vi "Helper Loop.vi"(8 "error in (no error)":errorcluster, 11 "Helper Loop in":refnum<class "Helper Loop.lvclass">) -> (0 "error out":errorcluster, 3 "Helper Loop out":refnum<class "Helper Loop.lvclass">)   [LabVIEW 2024, in "Helper Loop.lvlib" / "Helper Loop.lvclass"]
uses:
  Helper Loop.lvclass
  Helper Loop.lvclass/Helper Loop.ctl
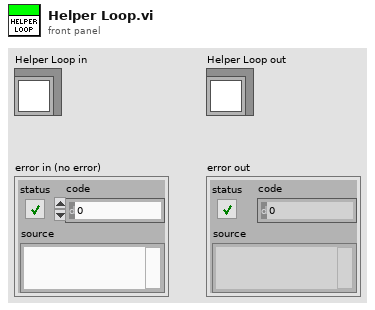
[diagram p1: front panel]
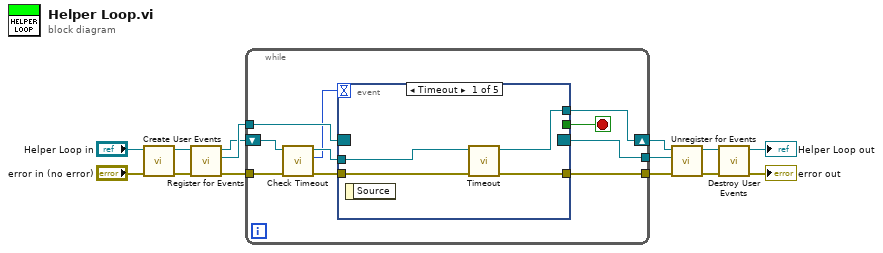
[diagram p0: block diagram]
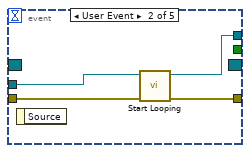
[diagram p2: hidden frame]
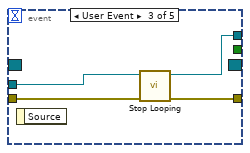
[diagram p3: hidden frame]
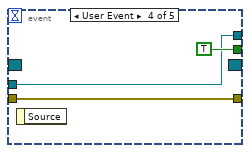
[diagram p4: hidden frame]
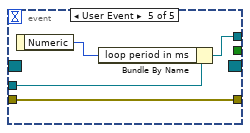
[diagram p5: hidden frame]
diagram:
  n1 = call-dynamic "Create User Events.vi"("error in (no error)"="error in (no error)", "Helper Loop in"="Helper Loop in") -> ("error out"=w11:errorcluster, "Helper Loop out"=w12:refnum<class "Helper Loop.lvclass">)  [unwired: 8 in]
  n2 = call-dynamic "Register for Events.vi"("error in (no error)"=w11, "Helper Loop in"=w12) -> ("error out"=w8:errorcluster, "event registration refnum"=w10:refnum<event-registration>, "Helper Loop out"=w9:refnum<class "Helper Loop.lvclass">)  [unwired: 7 in]
  n3 = while {
    shift-right: [w24] -> w5
    shift-left: w9 -> [w19]
    tunnel: w10 -> [w20]
    tunnel: [w22] -> w2
    tunnel: w8 -> [w18]
    tunnel: [w21] -> w1
    stop <- w23 stop-if-true
    n4 = call-dynamic "Check Timeout.vi"("error in (no error)"=w18, "Helper Loop in"=w19) -> ("error out"=w15:errorcluster, "timeout"=w16:i32, "Helper Loop out"=w17:refnum<class "Helper Loop.lvclass">)  [unwired: 7 in]
    n5 = event shown="[0] Timeout" {
      selector: w20 -> [_ _ _ _ _]
      dyn-events: [_ _ _ _ _] -> w21
      timeout: w16 -> [_ _ _ _ _]
      tunnel: [w27 w29 w33 w38 w41] -> w24
      tunnel: w17 -> [w28 w32 w36 w38 w43]
      tunnel: [_ _ _ TRUE _] -> w23
      tunnel: [w26 w30 w34 w37 w40] -> w22
      tunnel: w15 -> [w25 w31 w35 w37 w40]
      event Timeout {
        n6 = event-data() -> ()  [unwired: 1 in, 1 out]
        n7 = call-dynamic "Timeout.vi"("error in (no error)"=w25, "Helper Loop in"=w28) -> ("error out"=w26:errorcluster, "Helper Loop out"=w27:refnum<class "Helper Loop.lvclass">)  [unwired: 8 in]
      }
      event User Event {
        n8 = event-data() -> ()  [unwired: 1 in, 1 out]
        n9 = call-dynamic "Start Looping.vi"("error in (no error)"=w31, "Helper Loop in"=w32) -> ("error out"=w30:errorcluster, "Helper Loop out"=w29:refnum<class "Helper Loop.lvclass">)  [unwired: 8 in]
      }
      event User Event {
        n10 = event-data() -> ()  [unwired: 1 in, 1 out]
        n11 = call-dynamic "Stop Looping.vi"("error in (no error)"=w35, "Helper Loop in"=w36) -> ("error out"=w34:errorcluster, "Helper Loop out"=w33:refnum<class "Helper Loop.lvclass">)  [unwired: 8 in]
      }
      event User Event {
        n12 = event-data() -> ()  [unwired: 1 in, 1 out]
      }
      event User Event {
        n13 = event-data() -> ("Numeric"=w42:u32)  [unwired: 1 in]
        n14 = Bundle By Name(cluster=w43, "loop period in ms"=w42) -> (w41:refnum<class "Helper Loop.lvclass">)
      }
    }
  }
  n15 = call-dynamic "Unregister for Events.vi"("error in (no error)"=w2, "Event Registration Refnum"=w1, "Helper Loop in"=w5) -> ("error out"=w3:errorcluster, "Helper Loop out"=w4:refnum<class "Helper Loop.lvclass">)  [unwired: 7 in]
  n16 = call-dynamic "Destroy User Events.vi"("error in (no error)"=w3, "Helper Loop in"=w4) -> ("error out"=→"error out":errorcluster, "Helper Loop out"=→"Helper Loop out":refnum<class "Helper Loop.lvclass">)  [unwired: 8 in]
